vi "ODD_OR_EVEN.vi"() -> ()   [LabVIEW 2020]
panel:
  out "OUTPUT":string
  in  "N":dbl
  # "ODD OR EVEN"
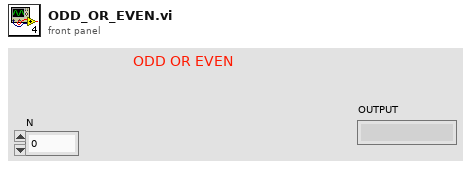
[diagram p1: front panel]
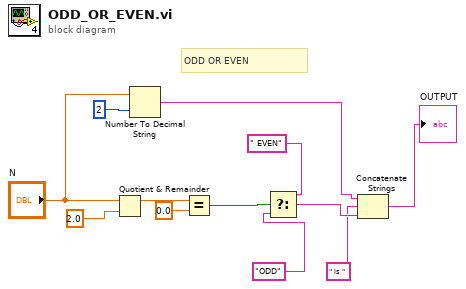
[diagram p0: block diagram]
diagram:
  # "ODD OR EVEN"
  n1 = Quotient & Remainder(x="N", y=2.0) -> (x-y*floor(x/y)=w11:dbl)  [unwired: 1 out]
  n2 = Number To Decimal String(number="N", width (-)=i16 2) -> (decimal integer string=w2:string)
  n3 = Equal?(x=w11, y=0.0) -> (x = y?=w9:bool)
  n4 = Select(t=" EVEN", s=w9, f="ODD") -> (s? t:f=w3:string)
  n5 = Concatenate Strings(w2, " is ", w3) -> (→"OUTPUT":string)
